vi "Plot_Many_Channels.vi"() -> (5 "Plug in titles":string[](array[string]), 7 "Plug in values":string[](array[string]))   [LabVIEW 2015]
uses:
  Globals/Meas_global.vi
panel:
  out "XY Graph":cluster{"Time (s)":dbl[], "Voltage":dbl[]}[](graph)
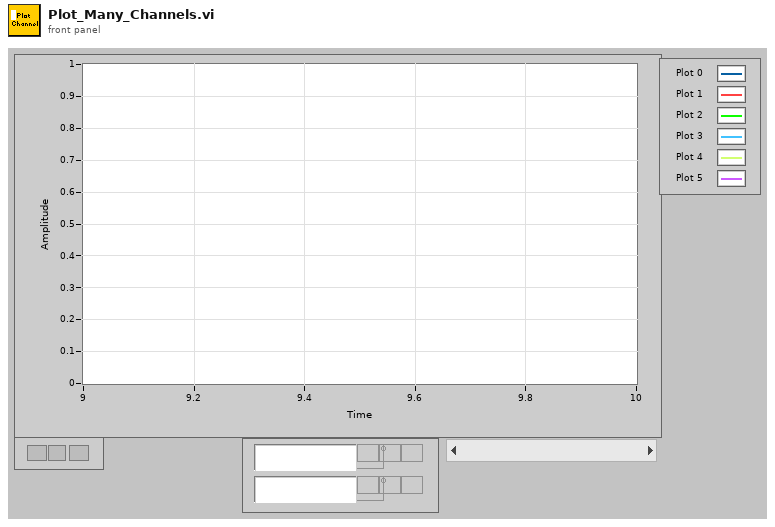
[diagram p1: front panel]
types:
  T1 = typedef "Time_Trace_Cluster.ctl" = cluster{"Weighting":dbl[], "Time (s)":dbl[], "Voltage":dbl[], "Eng Values":dbl[]}
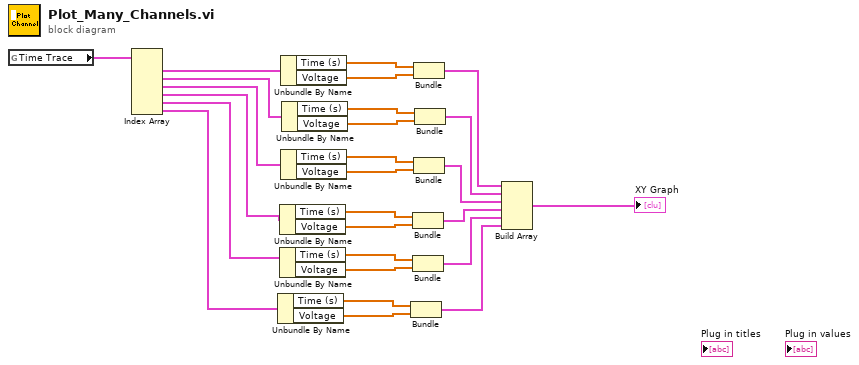
[diagram p0: block diagram]
diagram:
  n1 = global read "Meas_global.vi" "Time Trace"() -> (w16:T1[])
  n2 = Index Array(array=w16) -> (element #1=w17:T1, element #2=w9:T1, element #3=w8:T1, element #4=w6:T1, element #5=w5:T1, element #6=w7:T1)  [unwired: 6 in]
  n3 = Unbundle By Name(w7) -> ("Time (s)"=w11:dbl[], "Voltage"=w10:dbl[])
  n4 = Unbundle By Name(w6) -> ("Time (s)"=w15:dbl[], "Voltage"=w14:dbl[])
  n5 = Unbundle By Name(w5) -> ("Time (s)"=w12:dbl[], "Voltage"=w13:dbl[])
  n6 = Unbundle By Name(w17) -> ("Time (s)"=w20:dbl[], "Voltage"=w26:dbl[])
  n7 = Unbundle By Name(w8) -> ("Time (s)"=w18:dbl[], "Voltage"=w22:dbl[])
  n8 = Unbundle By Name(w9) -> ("Time (s)"=w19:dbl[], "Voltage"=w25:dbl[])
  n9 = Bundle("Time (s)"=w11, "Voltage"=w10) -> (w2:cluster{"Time (s)":dbl[], "Voltage":dbl[]})  [unwired: 1 in]
  n10 = Bundle("Time (s)"=w15, "Voltage"=w14) -> (w4:cluster{"Time (s)":dbl[], "Voltage":dbl[]})  [unwired: 1 in]
  n11 = Bundle("Time (s)"=w12, "Voltage"=w13) -> (w3:cluster{"Time (s)":dbl[], "Voltage":dbl[]})  [unwired: 1 in]
  n12 = Bundle("Time (s)"=w20, "Voltage"=w26) -> (w23:cluster{"Time (s)":dbl[], "Voltage":dbl[]})  [unwired: 1 in]
  n13 = Bundle("Time (s)"=w18, "Voltage"=w22) -> (w21:cluster{"Time (s)":dbl[], "Voltage":dbl[]})  [unwired: 1 in]
  n14 = Bundle("Time (s)"=w19, "Voltage"=w25) -> (w24:cluster{"Time (s)":dbl[], "Voltage":dbl[]})  [unwired: 1 in]
  n15 = Build Array(w23, w24, w21, w4, w3, w2) -> (→"XY Graph":cluster{"Time (s)":dbl[], "Voltage":dbl[]}[])
